vi "pmu_Map Phasor Phase.vi"(11 "phasor phase in":T1(ring)) -> (3 "phasor phase out":u8 format="%03b")   [LabVIEW 2013, in "NI_EP_PMU.lvlib"]
uses:
  <vilib>/addons/Electrical Power/PMU/NI_EP_PMU.lvlib
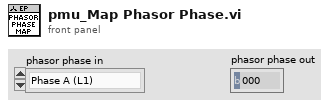
[diagram p1: front panel]
types:
  T1 = enum16{"Phase A (L1)", "Phase B (L2)", "Phase C (L3)", "Phase N", "Positive sequence", "Negative sequence", "Zero sequence"}
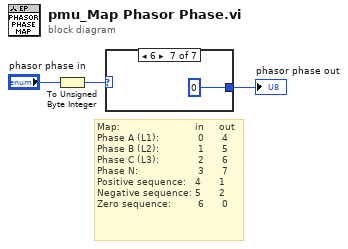
[diagram p0: block diagram]
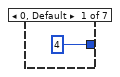
[diagram p2: hidden frame]
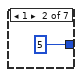
[diagram p3: hidden frame]
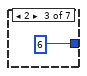
[diagram p4: hidden frame]
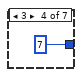
[diagram p5: hidden frame]
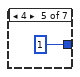
[diagram p6: hidden frame]
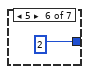
[diagram p7: hidden frame]
diagram:
  # "Map:                         in     out\nPhase A (L1):             0      4\nPhase B (L2):             1      5\nPhase C (L3):             2      6\nPhase N:                    3      7\nPositive sequence:   4      1\nNegative sequence: 5      2\nZero sequence:         6      0"
  n1 = To Unsigned Byte Integer(number="phasor phase in") -> (unsigned 8bit integer=w1:u8)
  n2 = case shown="6" w1 {
    tunnel: [u8 4 u8 5 u8 6 u8 7 u8 1 u8 2 u8 0] -> w2
    frame 0, Default {
    }
    frame 1 {
    }
    frame 2 {
    }
    frame 3 {
    }
    frame 4 {
    }
    frame 5 {
    }
    frame 6 {
    }
  }
  "phasor phase out" <- w2
